vi "Supply_SetVolts.vi"(8 "error in (no error)":errorcluster, 9 "Command string":string, 10 "Volts IN [V]":dbl, 11 "KE487 in":refnum<class "KE487.lvclass">) -> (0 "error out":errorcluster, 2 "Compliance exceeded?":bool, 3 "KE487 out":refnum<class "KE487.lvclass">)   [LabVIEW 2013, in "KE487.lvclass"]
uses:
  KE487.lvclass
  SupplyControl.lvclass
  InstrumentSetup.vi
  InstrControl.lvclass
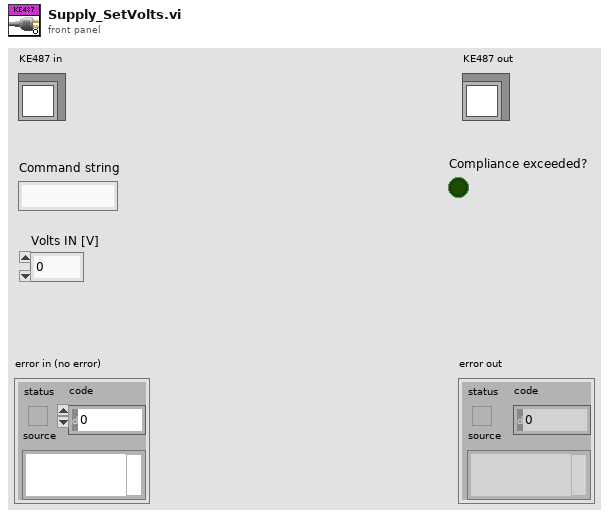
[diagram p1: front panel]
types:
  T1 = cluster{"Compliance":u16, "Range:":u16, "KE487":refnum<class "KE487.lvclass">}
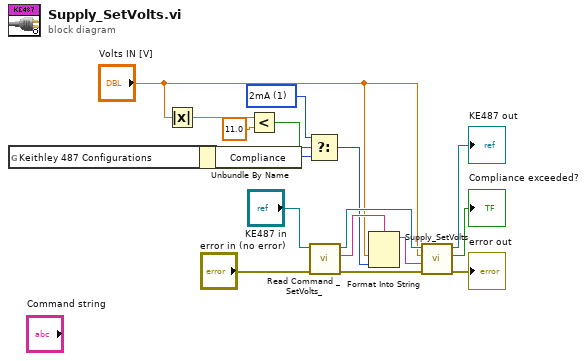
[diagram p0: block diagram]
diagram:
  w5 = u16 1 items=["20µA", "2mA"] ("Compliance")
  n1 = global read "InstrumentSetup.vi" "Keithley 487 Configurations"() -> (w14:T1)
  n2 = Absolute Value(x="Volts IN [V]") -> (abs(x)=w9:dbl)
  n3 = Unbundle By Name(w14) -> ("Compliance"=w6:u16)
  n4 = Less?(x=w9, y=11.0) -> (x < y?=w7:bool)
  n5 = Select(t=w5, s=w7, f=w6) -> (s? t:f=w3:u16)
  n6 = call-dynamic "Read Command _SetVolts_.vi"("error in (no error)"="error in (no error)", "SupplyControl in"="KE487 in") -> ("error out"=w1:errorcluster, "Command \"SetVolts\""=w11:string, "SupplyControl out"=w10:refnum<class "KE487.lvclass">)  [unwired: 7 in]
  n7 = Format Into String(format string=w11, "Volts IN [V]", w3) -> (resulting string=w4:string)  [unwired: 2 in, 1 out]
  n8 = call-parent "Supply_SetVolts.vi"("error in (no error)"=w1, "Command string"=w4, "Volts IN [V]"="Volts IN [V]", "SupplyControl in"=w10) -> ("error out"=→"error out":errorcluster, "Compliance exceeded?"=→"Compliance exceeded?":bool, "SupplyControl out"=→"KE487 out":refnum<class "KE487.lvclass">)  [unwired: 5 in]
